vi "AtDome_monitorCommand_closeShutter.vi"(8 "error in (no error)":errorcluster, 11 "command_closeShutter_Ctl":T1={"device"="", "property"="                                ", "action"="                                ", "itemValue"="                                ", "close"=FALSE}) -> (0 "error out":errorcluster, 2 "function return":i32, 3 "command_closeShutter_Ctl out":T1={"device"="", "property"="                                ", "action"="                                ", "itemValue"="                                ", "close"=FALSE})   [LabVIEW 2016, in "SALLV_AtDome.lvlib"]
doc: "int AtDome_shm_monitorCommand_closeShutterLV(AtDome_command_closeShutterLV *command_closeShutter_Ctl );"
uses:
  SALLV_AtDome.lvlib
  DataTypes/command_closeShutter.ctl
  SALLV_AtDome.so
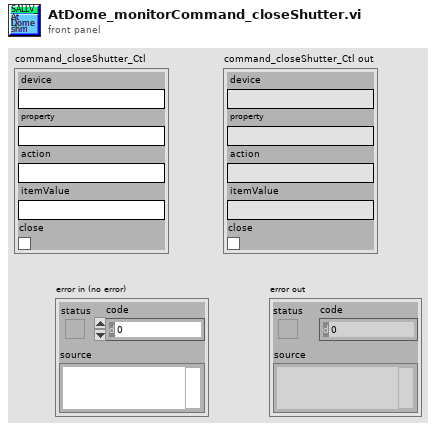
[diagram p1: front panel]
types:
  T1 = typedef "SALLV_AtDome.lvlib/command_closeShutter.ctl" = cluster{"device":string, "property":string, "action":string, "itemValue":string, "close":bool}
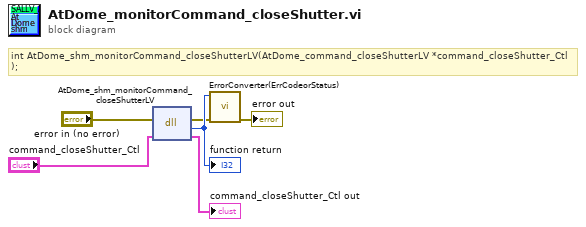
[diagram p0: block diagram]
diagram:
  # "int AtDome_shm_monitorCommand_closeShutterLV(AtDome_command_closeShutterLV *command_closeShutter_Ctl );"
  n1 = dll-call lib="home/andres/Desktop/SAL_AtDome/SALLV_AtDome.*" fn="AtDome_shm_monitorCommand_closeShutterLV"(error in="error in (no error)", "command_closeShutter_Ctl"="command_closeShutter_Ctl") -> (error out=w2:errorcluster, w6:i32, "command_closeShutter_Ctl"=→"command_closeShutter_Ctl out":T1)  [unwired: 2 in, 1 out]
  "function return" <- w6
  n2 = call "ErrorConverter(ErrCodeorStatus).vi"("error in (no error)"=w2, "error code"=w6) -> ("error out"=→"error out":errorcluster)  [unwired: 9 in]
